vi "GenerateSinWaveforms.vi"(6 "sampling info":cluster{"Fs":dbl, "#s":dbl}, 10 "amplitude":dbl, 11 "frequency":dbl) -> (3 "Waveform":waveform(dbl))   [LabVIEW 2019]
panel:
  out "Waveform Graph":waveform(dbl)(graph)
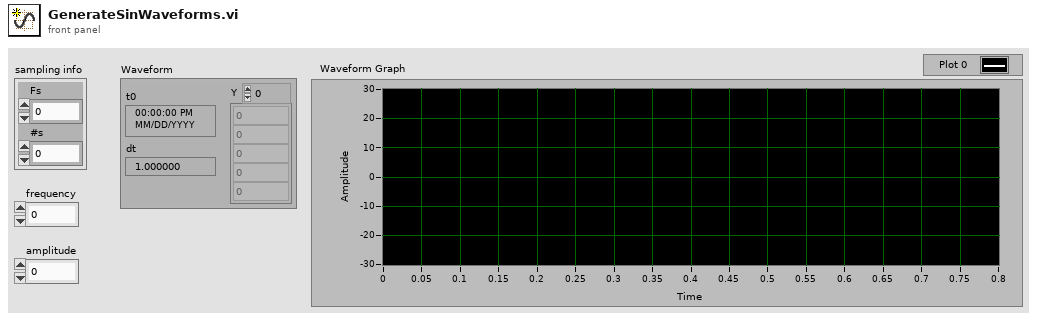
[diagram p1: front panel]
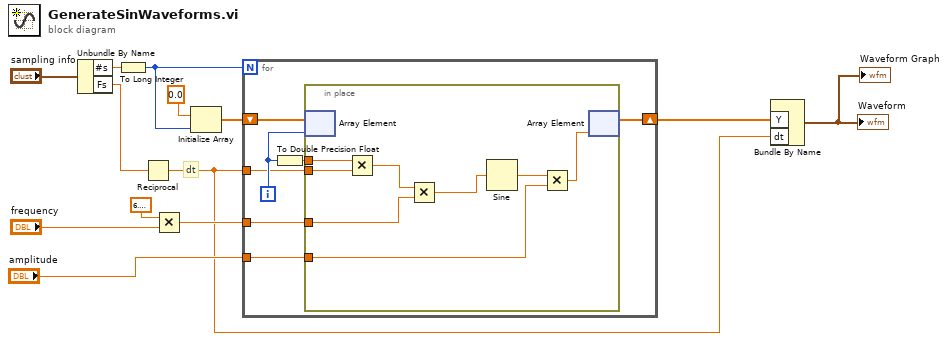
[diagram p0: block diagram]
diagram:
  # "dt"
  n1 = Unbundle By Name("sampling info") -> ("#s"=w4:dbl, "Fs"=w7:dbl)
  n2 = To Long Integer(number=w4) -> (32bit integer=w5:i32)
  n3 = Reciprocal(x=w7) -> (1/x=w9:dbl)
  n4 = Multiply(x=6.283185307179586, y="frequency") -> (x*y=w13:dbl)
  n5 = Initialize Array(0.0, w5) -> (w6:dbl[])
  n6 = for {
    N: w5 -> [_]
    shift-right: [w19] -> w8
    shift-left: w6 -> [w20]
    tunnel: w9 -> [w17]
    tunnel: w13 -> [w15]
    tunnel: "amplitude" -> [w14]
    i -> [w18]
    n7 = To Double Precision Float(number=w18) -> (double precision float=w16:dbl)
    n8 = in-place {
      in-place-border: w16 -> [w28]
      in-place-border: w17 -> [w27]
      in-place-border: w15 -> [w26]
      in-place-border: w14 -> [w23]
      n9 = in-place-array #1(w20, w18) -> ()  [unwired: 1 out]
      n10 = Multiply(x=w28, y=w27) -> (x*y=w22:dbl)
      n11 = Multiply(x=w22, y=w26) -> (x*y=w21:dbl)
      n12 = Sine(x=w21) -> (sin(x)=w25:dbl)
      n13 = Multiply(x=w25, y=w23) -> (x*y=w24:dbl)
      n14 = in-place-array #1(w24) -> (w19:dbl[])  [unwired: 1 out]
    }
  }
  n15 = Bundle By Name("Y"=w8, "dt"=w9) -> (→"Waveform" →"Waveform Graph":waveform(dbl))  [unwired: 1 in]
